vi "Add Subaddress.vi"(8 "error in":errorcluster, 10 "subaddress":T1, 11 "remote terminal in":T2 format="%.0x") -> (0 "error out":errorcluster, 2 "subaddress ref":T2 format="%.0x", 3 "remote terminal in":T2 format="%.0x")   [LabVIEW 2020, in "AIM MIL-STD-1553 Scripting.lvlib"]
uses:
  AIM MIL-STD-1553 Scripting.lvlib
  <vilib>/NI VeriStand/Custom Device API/Custom Device API.lvlib
  Constants.vi
  <vilib>/NI VeriStand/Custom Device API/Custom Device Item Ref.ctl
  Shared/Address.ctl
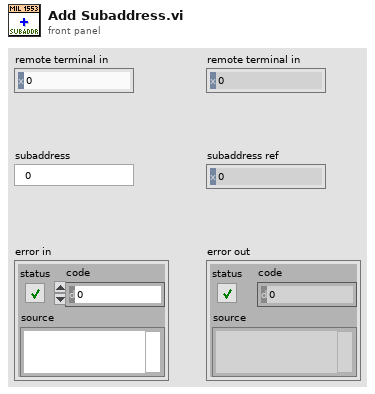
[diagram p1: front panel]
types:
  T1 = typedef "Address.ctl" = u16
  T2 = typedef "Custom Device API.lvlib/Custom Device Item Ref.ctl" = u64
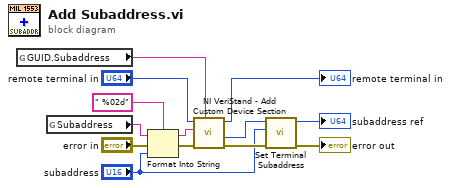
[diagram p0: block diagram]
diagram:
  n1 = global read "Constants.vi" "GUID.Subaddress"() -> (w13:string)
  n2 = global read "Constants.vi" "Subaddress"() -> (w3:string)
  n3 = Format Into String(format string=" %02d", initial string=w3, error in="error in", "subaddress") -> (resulting string=w6:string, error out=w4:errorcluster)
  n4 = call <vilib>:"NI VeriStand - Add Custom Device Section.vi"("GUID (Default Section)"=w13, "error in (no error)"=w4, "Section Name"=w6, "Parent Ref in"="remote terminal in") -> ("error out"=w9:errorcluster, "Section Ptr"=w2:T2, "Parent Ref out"=→"remote terminal in":T2)  [unwired: 4 in, 1 out]
  n5 = call "Set Terminal Subaddress.vi"("error in"=w9, "subaddress"="subaddress", "subaddress in"=w2) -> ("error out"=→"error out":errorcluster, "subaddress out"=→"subaddress ref":T2)  [unwired: 7 in]
